vi "Create All Message Queues.vi"(8 "error in (no error)":errorcluster, 10 "Master Queue In":refnum<queue>, 11 "Stand alone?":bool) -> (0 "error out":errorcluster, 3 "Message Queues out":T1)   [LabVIEW 2013, in "Cal Inst Message Queue.lvlib"]
doc: "This VI creates and initializes all the message queues for your application. If your application requires more than one message queue, right-click the \"Message Queues\" constant above and select Open Type Def. Add the new Message Queue(s) to the type definition, then initialize them in this VI."
uses:
  Cal Inst Message Queue.lvlib
  All Message Queues.ctl
  Message Cluster.ctl
  Enqueue Message (Single).vi
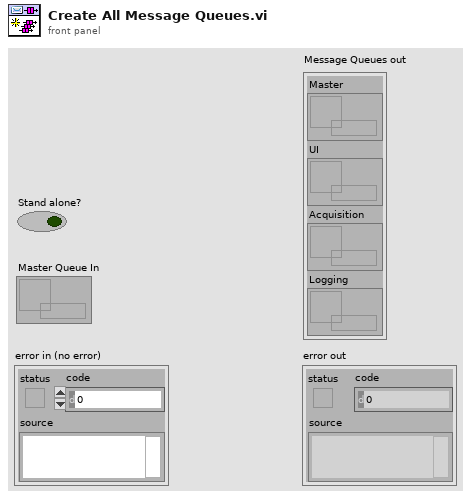
[diagram p1: front panel]
types:
  T1 = typedef "Cal Inst Message Queue.lvlib/All Message Queues.ctl" = cluster{"Master":refnum<queue>, "UI":refnum<queue>, "Acquisition":refnum<queue>, "Logging":refnum<queue>}
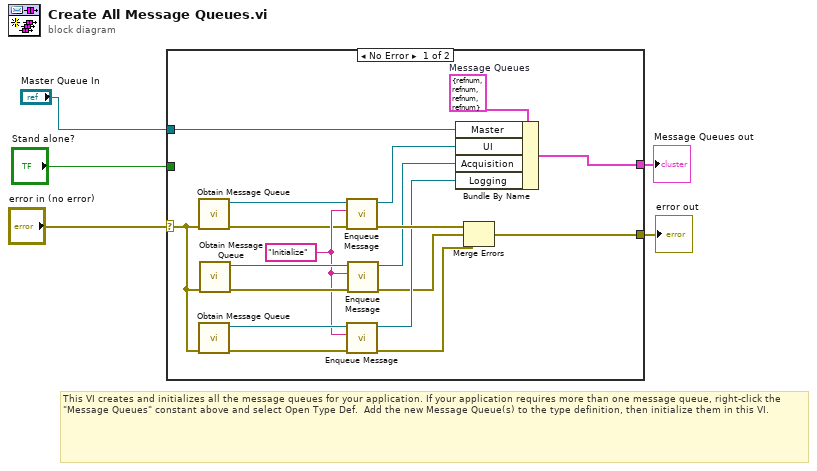
[diagram p0: block diagram]
diagram:
  # "This VI creates and initializes all the message queues for your application. If your application requires more than one message queue, right-click the \"Message Queues\" constant above and select Open Type Def.  Add the new Message Queue(s) to the type definition, then initialize them in this VI."
  n1 = case shown="No Error" "error in (no error)" {
    selector: "error in (no error)" -> [w16 w24]
    tunnel: [w11 w24] -> w5
    tunnel: [w21 _] -> w4
    tunnel: "Stand alone?" -> [_ _]
    tunnel: "Master Queue In" -> [w8 _]
    frame No Error {
      w15 = "Initialize" ("Message")
      w22 = T1 {"Master"=refnum, "UI"=refnum, "Acquisition"=refnum, "Logging"=refnum}  # Message Queues
      n2 = call "Obtain Message Queue.vi"("error in (no error)"=w16) -> ("error out"=w7:errorcluster, "Message Queue"=w6:refnum<queue>)  [unwired: 9 in]
      n3 = call "Obtain Message Queue.vi"("error in (no error)"=w16) -> ("error out"=w18:errorcluster, "Message Queue"=w17:refnum<queue>)  [unwired: 9 in]
      n4 = call "Obtain Message Queue.vi"("error in (no error)"=w16) -> ("error out"=w19:errorcluster, "Message Queue"=w20:refnum<queue>)  [unwired: 9 in]
      n5 = call-poly "Enqueue Message.vi"("error in (no error)"=w7, "Message"=w15, "Message Queue"=w6) -> ("error out"=w23:errorcluster, "dup Message Queue"=w14:refnum<queue>)  [unwired: 7 in]
      n6 = call-poly "Enqueue Message.vi"("error in (no error)"=w18, "Message"=w15, "Message Queue"=w17) -> ("error out"=w9:errorcluster, "dup Message Queue"=w12:refnum<queue>)  [unwired: 7 in]
      n7 = call-poly "Enqueue Message.vi"("error in (no error)"=w19, "Message"=w15, "Message Queue"=w20) -> ("error out"=w10:errorcluster, "dup Message Queue"=w13:refnum<queue>)  [unwired: 7 in]
      n8 = Bundle By Name(cluster=w22, "Master"=w8, "UI"=w14, "Acquisition"=w13, "Logging"=w12) -> (w21:T1)
      n9 = Merge Errors(w23, w10, w9) -> (w11:errorcluster)
    }
    frame Error {
    }
  }
  "Message Queues out" <- w4
  "error out" <- w5
